vi "Create Method Metadata.vi"(8 "error in (no error)":errorcluster, 11 "services":u64[](array[numeric])) -> (0 "error out":errorcluster, 3 "Method Parameters":T1[](array[typedef]))   [LabVIEW 2019, in "gRPC Template Creation Utility.lvlib"]
uses:
  gRPC Template Creation Utility.lvlib
  TypeDefs/RPC Method Parameters.ctl
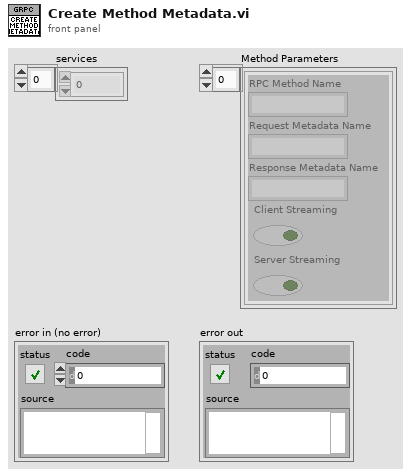
[diagram p1: front panel]
types:
  T1 = typedef "gRPC Template Creation Utility.lvlib/RPC Method Parameters.ctl" = cluster{"RPC Method Name":string, "Request Metadata Name":string, "Response Metadata Name":string, "Client Streaming":bool, "Server Streaming":bool}
  T2 = typedef "gRPC Template Creation Utility.lvlib/Message Metadata (Scripting).ctl" = cluster{"Version":i32, "Name":string, "Type Url":string, "Elements":T3[]}
  T3 = typedef "gRPC Template Creation Utility.lvlib/Message Element Metadata (Scripting).ctl" = cluster{"Field Name":string, "Embedded Message Name":string, "Protobuf Index":i32, "MessageElementType":T4, "Repeated":bool}
  T4 = typedef "gRPC Template Creation Utility.lvlib/Message Element Type.ctl" = enum32{"Int32Value", "FloatValue", "DoubleValue", "BoolValue", "StringValue", "MessageValue", "Int64Value", "UInt32Value", "UInt64Value", "EnumValue", "Bytes", "Fixed64", "Fixed32", "SFixed64", "SFixed32", "SInt64", "SInt32"}
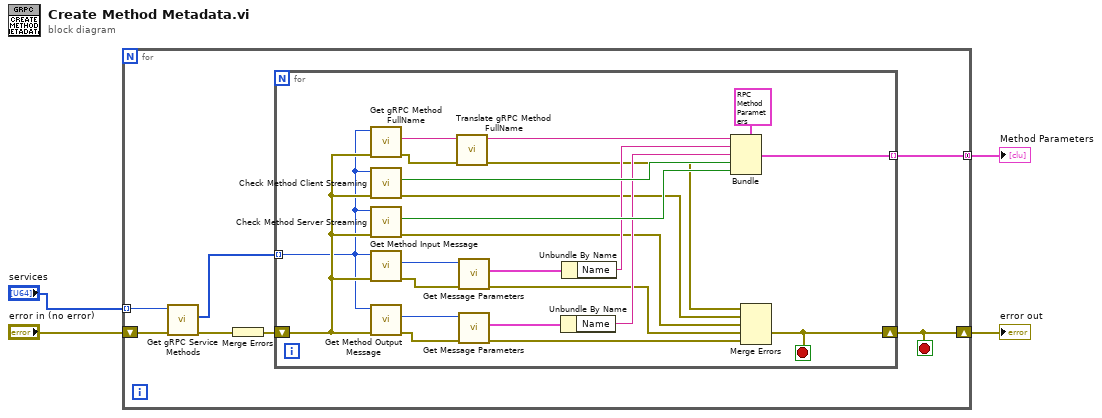
[diagram p0: block diagram]
diagram:
  n1 = for {
    tunnel: "services" -> [w11] mode=indexing
    tunnel: [w10] -> w2 mode=concatenating
    shift-right: [w5] -> w3
    shift-left: "error in (no error)" -> [w8]
    stop <- w5 stop-if-true
    n2 = call "Get gRPC Service Methods.vi"("error in (no error)"=w8, "Service ref in"=w11) -> ("error out"=w7:errorcluster, "Service Methods"=w9:u64[])  [unwired: 7 in, 1 out]
    n3 = Merge Errors(w7) -> (w6:errorcluster)
    n4 = for {
      tunnel: w9 -> [w16] mode=indexing
      tunnel: [w34] -> w10 mode=indexing
      shift-right: [w18] -> w5
      shift-left: w6 -> [w17]
      stop <- w18 stop-if-true
      n5 = call "Get gRPC Method FullName.vi"("error in (no error)"=w17, "Method ref in"=w16) -> ("error out"=w15:errorcluster, "Method Full Name"=w14:string)  [unwired: 7 in, 1 out]
      n6 = call "Check Method Client Streaming.vi"("error in (no error)"=w17, "Method ref in"=w16) -> ("error out"=w22:errorcluster, "is Client Streaming"=w33:bool)  [unwired: 7 in, 1 out]
      n7 = call "Check Method Server Streaming.vi"("error in (no error)"=w17, "Method ref in"=w16) -> ("error out"=w21:errorcluster, "is Server Streaming"=w32:bool)  [unwired: 7 in, 1 out]
      n8 = call "Get Method Input Message.vi"("error in (no error)"=w17, "Method ref in"=w16) -> ("error out"=w27:errorcluster, "Message ref out"=w30:u64)  [unwired: 7 in, 1 out]
      n9 = call "Get Method Output Message.vi"("error in (no error)"=w17, "Method ref in"=w16) -> ("error out"=w28:errorcluster, "Message ref out"=w29:u64)  [unwired: 7 in, 1 out]
      n10 = call "Translate gRPC Method FullName.vi"("error in (no error)"=w15, "Method Full Name in"=w14) -> ("error out"=w12:errorcluster, "Method Full Name out"=w13:string)  [unwired: 8 in]
      n11 = call "Get Message Parameters.vi"("error in (no error)"=w27, "Message ref in"=w30) -> ("error out"=w20:errorcluster, "Message Metadata"=w24:T2)  [unwired: 7 in, 1 out]
      n12 = call "Get Message Parameters.vi"("error in (no error)"=w28, "Message ref in"=w29) -> ("error out"=w19:errorcluster, "Message Metadata"=w23:T2)  [unwired: 7 in, 1 out]
      n13 = Unbundle By Name(w23) -> ("Name"=w25:string)
      n14 = Unbundle By Name(w24) -> ("Name"=w26:string)
      n15 = Bundle(cluster=T1 {"RPC Method Name"="/queryserver.QueryServer/Invoke", "Request Metadata Name"="InvokeRequest", "Response Metadata Name"="InvokeResponse", "Client Streaming"=FALSE, "Server Streaming"=FALSE}, "RPC Method Name"=w13, "Request Metadata Name"=w26, "Response Metadata Name"=w25, "Client Streaming"=w33, "Server Streaming"=w32) -> (w34:T1)
      n16 = Merge Errors(w12, w22, w21, w20, w19) -> (w18:errorcluster)
    }
  }
  "error out" <- w3
  "Method Parameters" <- w2
